vi "PythonIntegrate.vi"() -> ()   [LabVIEW 2018]
uses:
  <vilib>/Enthought/Python Integration Toolkit/api/Unpack Int.vi
  <vilib>/Enthought/Python Integration Toolkit/Python Integration Toolkit.lvlib
panel:
  in  "数值":dbl
  out "Value":i32
  in  "路径":path
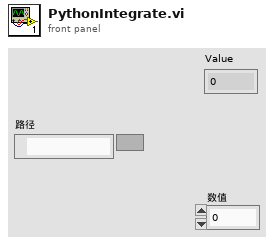
[diagram p1: front panel]
types:
  T1 = typedef "Python Integration Toolkit.lvlib/Session ID.ctl" = u64
  T2 = typedef "Python Integration Toolkit.lvlib/Python Objects.ctl" = variant
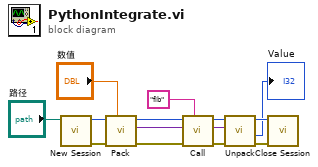
[diagram p0: block diagram]
diagram:
  n1 = call <vilib>:"New Session.vi"("Path to Python Module (.py File)"="路径") -> ("error out"=w6:errorcluster, "Session ID out"=w11:T1)  [unwired: 9 in]
  n2 = call <vilib>:"Pack.vi"("Argument"="数值", "error in (no error)"=w6, "Session ID"=w11) -> ("error out"=w14:errorcluster, "Python Object References Out"=w2:T2, "Session ID out"=w12:T1)  [unwired: 6 in]
  n3 = call <vilib>:"Call.vi"("Function or Method Name"="fib", "error in (no error)"=w14, "Python Object References In"=w2, "Session ID"=w12) -> ("error out"=w13:errorcluster, "Python Object References Out"=w3:T2, "Session ID out"=w10:T1)  [unwired: 5 in]
  n4 = call-poly <vilib>:"Unpack.vi"("error in (no error)"=w13, "Python Object References In"=w3, "Session ID"=w10) -> ("error out"=w8:errorcluster, "Value"=→"Value":i32, "Session ID out"=w9:T1)  [unwired: 5 in, 1 out]
  n5 = call <vilib>:"Close Session.vi"("error in (no error)"=w8, "Session ID"=w9) -> ()  [unwired: 9 in, 1 out]
